vi "Fetch Measurement (RJDJ).vi"(0 "VISA resource name":refnum<visa-resource-name>, 11 "error in (no error)":errorcluster) -> (3 "TJ":T1, 4 "VISA resource name out":refnum<visa-resource-name>, 6 "RJ":T1, 8 "DJ":T1, 10 "PJ":T2, 12 "DDJ":T1, 13 "DCD":cluster{"Result":dbl, "State":i32}, 14 "ISI":T1, 15 "error out":errorcluster)   [LabVIEW 2009, in "Agilent 8000 Series.lvlib"]
doc: "Returns the results of the RJDJ Jitter measurment."
uses:
  Agilent 8000 Series.lvlib
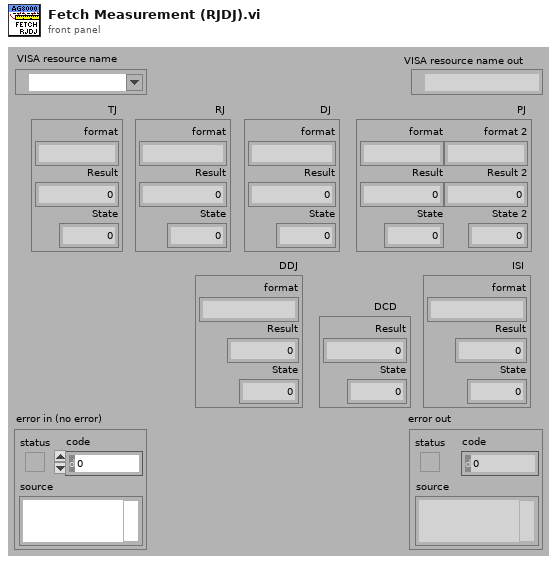
[diagram p1: front panel]
types:
  T1 = cluster{"format":string, "Result":dbl, "State":i32}
  T2 = cluster{"format":string, "Result":dbl, "State":i32, "format 2":string, "Result 2":dbl, "State 2":i32}
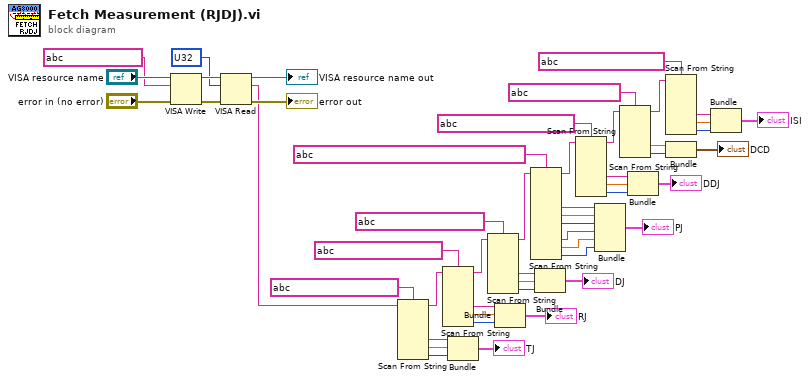
[diagram p0: block diagram]
diagram:
  n1 = VISA Write(VISA resource name="VISA resource name", write buffer=string ?, error in (no error)="error in (no error)") -> (VISA resource name out=w49:refnum<visa-resource-name>, error out=w48:errorcluster)  [unwired: 1 out]
  n2 = VISA Read(VISA resource name=w49, byte count=u32 ?, error in (no error)=w48) -> (VISA resource name out=→"VISA resource name out":refnum<visa-resource-name>, read buffer=w2:string, error out=→"error out":errorcluster)  [unwired: 1 out]
  n3 = Scan From String(format string=string ?, input string=w2) -> (remaining string=w40:string, output 2=w31:string, output 3=w30:dbl, output 4=w29:i32)  [unwired: 7 in, 2 out]
  n4 = Scan From String(format string=string ?, input string=w40) -> (remaining string=w44:string, output 2=w27:string, output 3=w26:dbl, output 4=w25:i32)  [unwired: 7 in, 2 out]
  n5 = Bundle(w31, w30, w29) -> (→"TJ":cluster{string, dbl, i32})  [unwired: 1 in]
  n6 = Scan From String(format string=string ?, input string=w44) -> (remaining string=w43:string, output 2=w24:string, output 3=w23:dbl, output 4=w22:i32)  [unwired: 7 in, 2 out]
  n7 = Bundle(w27, w26, w25) -> (→"RJ":cluster{string, dbl, i32})  [unwired: 1 in]
  n8 = Scan From String(format string=string ?, input string=w43) -> (remaining string=w42:string, output 2=w20:string, output 3=w19:dbl, output 4=w18:i32, output 6=w17:string, output 7=w16:dbl, output 8=w15:i32)  [unwired: 12 in, 2 out]
  n9 = Bundle(w24, w23, w22) -> (→"DJ":cluster{string, dbl, i32})  [unwired: 1 in]
  n10 = Scan From String(format string=string ?, input string=w42) -> (remaining string=w41:string, output 2=w13:string, output 3=w12:dbl, output 4=w11:i32)  [unwired: 7 in, 2 out]
  n11 = Bundle(w20, w19, w18, w17, w16, w15) -> (→"PJ":cluster{string, dbl, i32, string, dbl, i32})  [unwired: 1 in]
  n12 = Scan From String(format string=string ?, input string=w41) -> (remaining string=w39:string, output 2=w9:dbl, output 3=w8:i32)  [unwired: 6 in, 2 out]
  n13 = Bundle(w13, w12, w11) -> (→"DDJ":cluster{string, dbl, i32})  [unwired: 1 in]
  n14 = Scan From String(format string=string ?, input string=w39) -> (output 2=w6:string, output 3=w5:dbl, output 4=w4:i32)  [unwired: 7 in, 3 out]
  n15 = Bundle(w9, w8) -> (→"DCD":cluster{dbl, i32})  [unwired: 1 in]
  n16 = Bundle(w6, w5, w4) -> (→"ISI":cluster{string, dbl, i32})  [unwired: 1 in]
